vi "Configure Scan Interval.vi"(7 "Hours":i8 min=0 max=99 step=1, 8 "error in (no error)":errorcluster, 9 "Seconds":i8 min=0 max=99 step=1, 10 "Minutes":i8 min=0 max=99 step=1, 11 "VISA resource name":refnum<visa-resource-name>) -> (0 "error out":errorcluster, 3 "VISA resource name out":refnum<visa-resource-name>)   [LabVIEW 2013, in "Fluke 2625A.lvlib"]
uses:
  <instrlib>/Fluke 2625A/Fluke 2625A.lvlib
panel:
  out "concatenated string":string
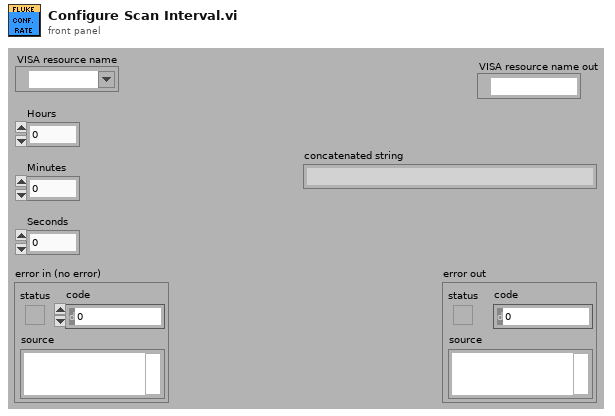
[diagram p1: front panel]
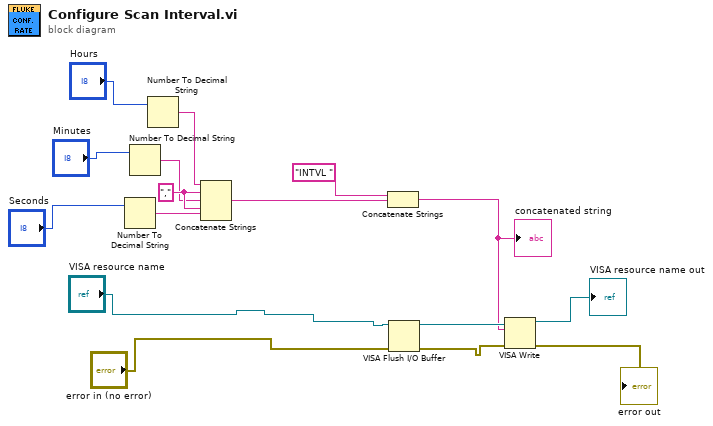
[diagram p0: block diagram]
diagram:
  w9 = "," ("string")
  n1 = Number To Decimal String(number="Seconds") -> (decimal integer string=w6:string)  [unwired: 1 in]
  n2 = Number To Decimal String(number="Minutes") -> (decimal integer string=w7:string)  [unwired: 1 in]
  n3 = Number To Decimal String(number="Hours") -> (decimal integer string=w8:string)  [unwired: 1 in]
  n4 = Concatenate Strings(w8, w9, w7, w9, w6) -> (w3:string)
  n5 = Concatenate Strings("INTVL ", w3) -> (w11:string)
  "concatenated string" <- w11
  n6 = VISA Flush I/O Buffer(VISA resource name="VISA resource name", error in (no error)="error in (no error)") -> (VISA resource name out=w16:refnum<visa-resource-name>, error out=w15:errorcluster)  [unwired: 1 in]
  n7 = VISA Write(VISA resource name=w16, write buffer=w11, error in (no error)=w15) -> (VISA resource name out=→"VISA resource name out":refnum<visa-resource-name>, error out=→"error out":errorcluster)  [unwired: 1 out]
